vi "Pre Launch Init.vi"(11 "Host MSS Test Actor in":refnum<class "Host MSS Test Actor.lvclass">) -> (0 "error out":errorcluster, 3 "Host MSS Test Actor out":refnum<class "Host MSS Test Actor.lvclass">)   [LabVIEW 2023, in "Host MSS Test Actor.lvlib" / "Host MSS Test Actor.lvclass"]
doc: "(<B>Filename</B>: Actor Framework.lvlib:Actor.lvclass:Pre Launch Init.vi)\n\nDefines behavior that occurs after the Launch Nested Actor method is invoked but before the actor's Actor Core method begins running.\n\nBy default, this method does nothing. A descendant class may override it to define behavior."
uses:
  Host MSS Test Actor.lvclass
  <vilib>/ActorFramework/Actor/Actor.lvclass
  Host MSS Test Actor.lvclass/Host MSS Test Actor.ctl
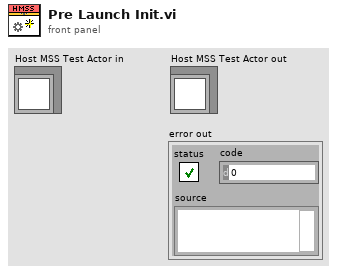
[diagram p1: front panel]
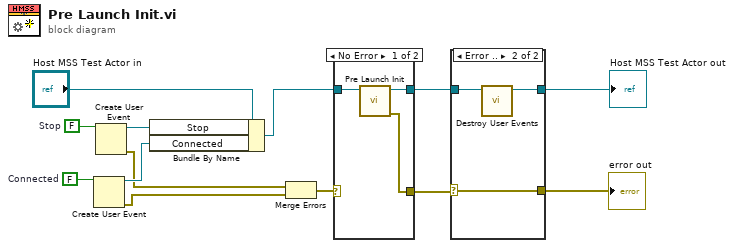
[diagram p0: block diagram]
diagram:
  w2 = FALSE  # Connected
  w3 = FALSE  # Stop
  n1 = Create User Event(user event datatype=w2) -> (user event=w12:refnum<user-event>, error out=w10:errorcluster)  [unwired: 1 in]
  n2 = Create User Event(user event datatype=w3) -> (user event=w13:refnum<user-event>, error out=w11:errorcluster)  [unwired: 1 in]
  n3 = Bundle By Name(cluster="Host MSS Test Actor in", "Stop"=w13, "Connected"=w12) -> (w1:refnum<class "Host MSS Test Actor.lvclass">)
  n4 = Merge Errors(w11, w10) -> (w9:errorcluster)
  n5 = case shown="No Error" w9 {
    selector: w9 -> [_ w17]
    tunnel: w1 -> [w16 w18]
    tunnel: [w15 w17] -> w7
    tunnel: [w14 w18] -> w5
    frame No Error {
      n6 = call-parent "Pre Launch Init.vi"("Actor in"=w16) -> ("error out"=w15:errorcluster, "Actor out"=w14:refnum<class "Host MSS Test Actor.lvclass">)  [unwired: 9 in]
    }
    frame Error {
    }
  }
  n7 = case shown="Error .." w7 {
    selector: w7 -> [w20 w23]
    tunnel: [w20 w23] -> w6
    tunnel: w5 -> [w19 w22]
    tunnel: [w19 w21] -> w4
    frame No Error {
    }
    frame Error {
      n8 = call "Destroy User Events.vi"("Host MSS Test Actor in"=w22) -> ("Host MSS Test Actor out"=w21:refnum<class "Host MSS Test Actor.lvclass">)  [unwired: 10 in]
    }
  }
  "error out" <- w6
  "Host MSS Test Actor out" <- w4
